vi "System.vi"(0 "Setup in":T6={"No.VI"=0, "Category"="", "StepName"="", "Seq setup flattened"="", "Comment"="", "Steps config."=[], "Jump config"=[], "Start"=0.0, "Increment"=0.0, "Name"="Pa", "Unit"="Pa", "Y data"=1, "Y prefix"="", "Y dB ref"=1.0, "Y unit"="", "Repeat State Array"=[]} {"Repeat State Array"."Start" format="%#_5g"; "Y dB ref" format="%.1f"; "Y data" items=["dB", "Lin"]; "Start" format="%#_5g"}, 5 "Data in":T4 {"Z data" items=["dB", "Lin"]; "X data" items=["dB", "Lin"]; "Y data" items=["dB", "Lin"]; "Z dB ref" format="%.1f"; "Z axis" items=["Log", "Lin"]; "X dB ref" format="%.1f"; "X axis" items=["Log", "Lin"]; "Y axis" items=["Log", "Lin"]; "Y dB ref" format="%.1f"; "Curve"."z" format="%.2f"; "Curve"."y" format="%.2f"; "Curve"."x" format="%.2f"}, 7 "Results in":T2 {"Margin" format="%.2f"}, 9 "Seq Setup in":string, 11 "Step name":string, 12 "Hardware in":string, 13 "Calibration in":string) -> (3 "Types Out":string[](array[string]), 4 "Inserted Names Out":string[](array[string]), 6 "Data out":T4 {"Z data" items=["dB", "Lin"]; "X data" items=["dB", "Lin"]; "Y data" items=["dB", "Lin"]; "Z dB ref" format="%.1f"; "Z axis" items=["Log", "Lin"]; "X dB ref" format="%.1f"; "X axis" items=["Log", "Lin"]; "Y axis" items=["Log", "Lin"]; "Y dB ref" format="%.1f"; "Curve"."z" format="%.2f"; "Curve"."y" format="%.2f"; "Curve"."x" format="%.2f"}, 8 "Results out":T2 {"Margin" format="%.2f"}, 10 "Wave out":T1[](array[typedef]) {"Y dB ref" format="%.1f"; "Y axis" items=["Log", "Lin"]; "Y data" items=["dB", "Lin"]; "X data" items=["dB", "Lin"]})   [LabVIEW 2013]
uses:
  CRYCustom and Run Seq.llb/CRYData Cluster Array.ctl
  CRYCustom and Run Seq.llb/CRYData Cluster.ctl
  CRYCustom and Run Seq.llb/CRYResult Cluster Array.ctl
  CRYCustom and Run Seq.llb/CRYResult Cluster.ctl
  CRYCustom and Run Seq.llb/CRYStep.ctl
  CRYCustom and Run Seq.llb/CRYWaveform Cluster.ctl
panel:
  in  "error in (no error)":errorcluster
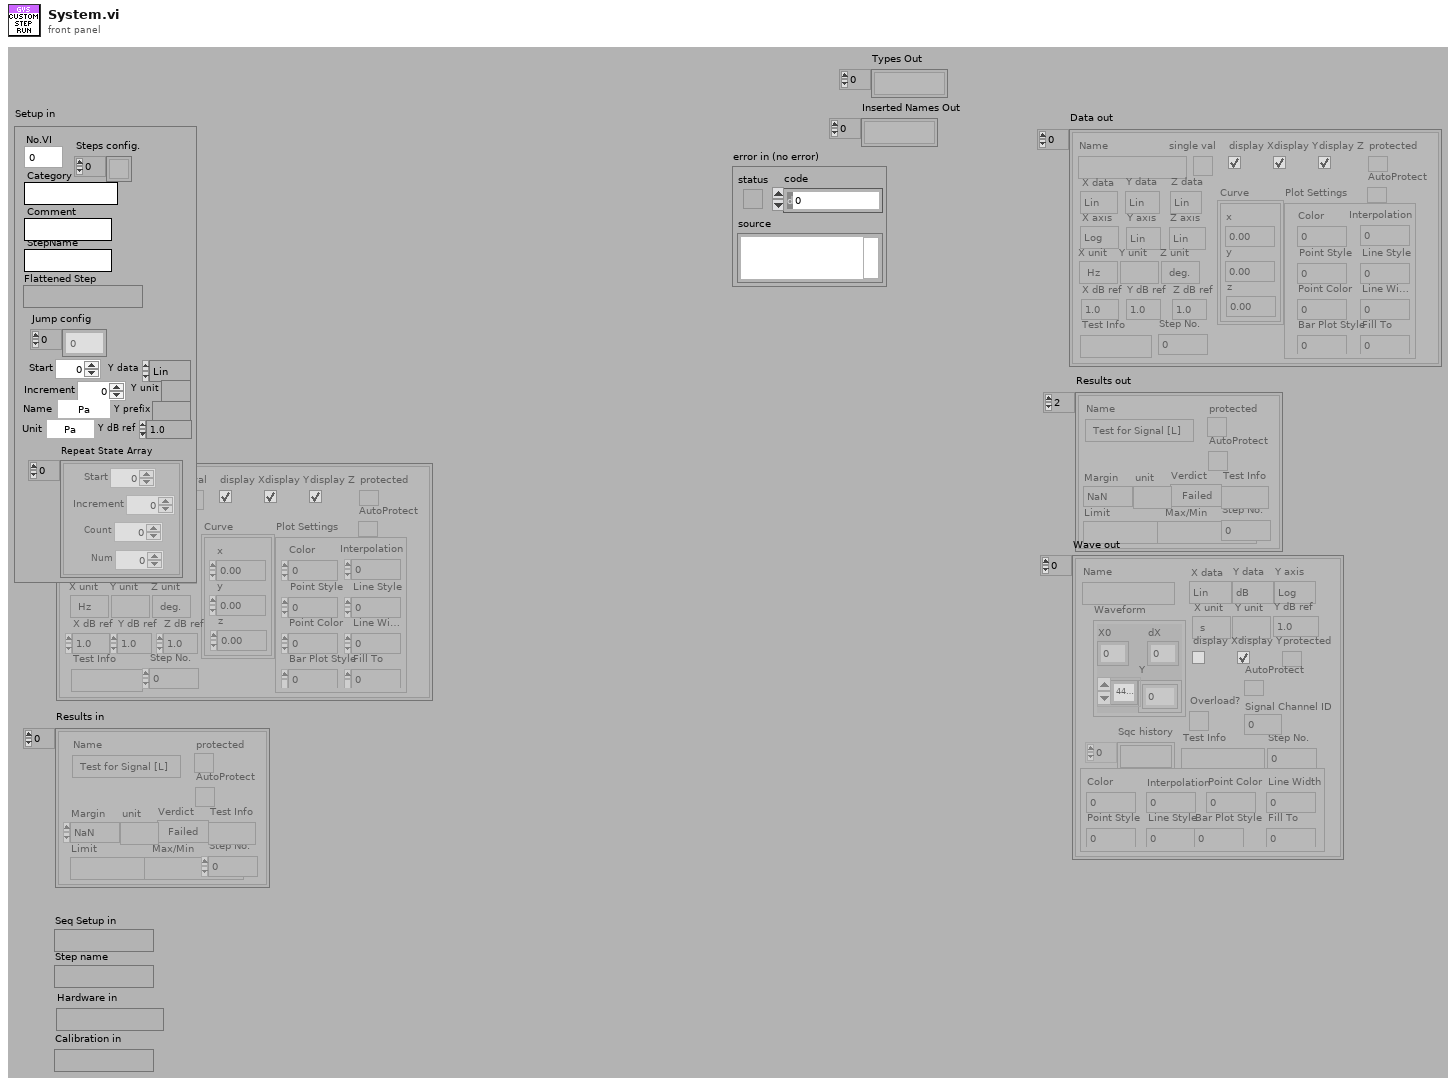
[diagram p1: front panel]
types:
  T1 = typedef "CRYWaveform Cluster.ctl" = cluster{"Waveform":cluster{"X0":dbl, "dX":dbl, "Y":sgl[]}, "X data":u16, "Y data":u16, "Y axis":u16, "X unit":string, "Y unit":string, "Y dB ref":dbl, "display Y":bool, "display X":bool, "Overload?":bool, "Test Info":string, "Step No.":i32, "Name":string, "protected":bool, "Sqc history":string[], "Signal Channel ID":i32, "Plot Settings":cluster{"Color":u32, "Interpolation":u8, "Point Style":u8, "Line Style":u8, "Point Color":u32, "Line Width":u8, "Bar Plot Style":u8, "Fill To":i16}, "AutoProtect":bool}
  T2 = typedef "CRYResult Cluster Array.ctl" = T3[]
  T3 = typedef "CRYResult Cluster.ctl" = cluster{"Name":string, "Margin":dbl, "unit":string, "Verdict":bool, "Limit":string, "Max/Min":string, "protected":bool, "Step No.":i32, "Test Info":string, "AutoProtect":bool}
  T4 = typedef "CRYData Cluster Array.ctl" = T5[]
  T5 = typedef "CRYData Cluster.ctl" = cluster{"Name":string, "Curve":cluster{"x":dbl, "y":dbl, "z":dbl}[], "X data":u16, "Y data":u16, "Z data":u16, "X axis":u16, "Y axis":u16, "Z axis":u16, "X unit":string, "Y unit":string, "Z unit":string, "X dB ref":dbl, "Y dB ref":dbl, "Z dB ref":dbl, "single val":bool, "protected":bool, "display X":bool, "display Y":bool, "display Z":bool, "Test Info":string, "Step No.":i32, "Plot Settings":cluster{"Color":u32, "Interpolation":u8, "Point Style":u8, "Line Style":u8, "Point Color":u32, "Line Width":u8, "Bar Plot Style":u8, "Fill To":i16}, "AutoProtect":bool}
  T6 = typedef "CRYStep.ctl" = cluster{"No.VI":i32, "Category":string, "StepName":string, "Seq setup flattened":string, "Comment":string, "Steps config.":bool[], "Jump config":i32[], "Start":dbl, "Increment":dbl, "Name":string, "Unit":string, "Y data":u16, "Y prefix":string, "Y dB ref":dbl, "Y unit":string, "Repeat State Array":cluster{"Start":dbl, "Increment":dbl, "Count":i32, "Num":i32}[]}
  T7 = cluster{"Command Line":string, "Working Directory":path, "WaitForCompletion":bool}
  T8 = typedef "CRYCustom Cluster.ctl" = cluster{"Help":string, "Flatten Data":string}
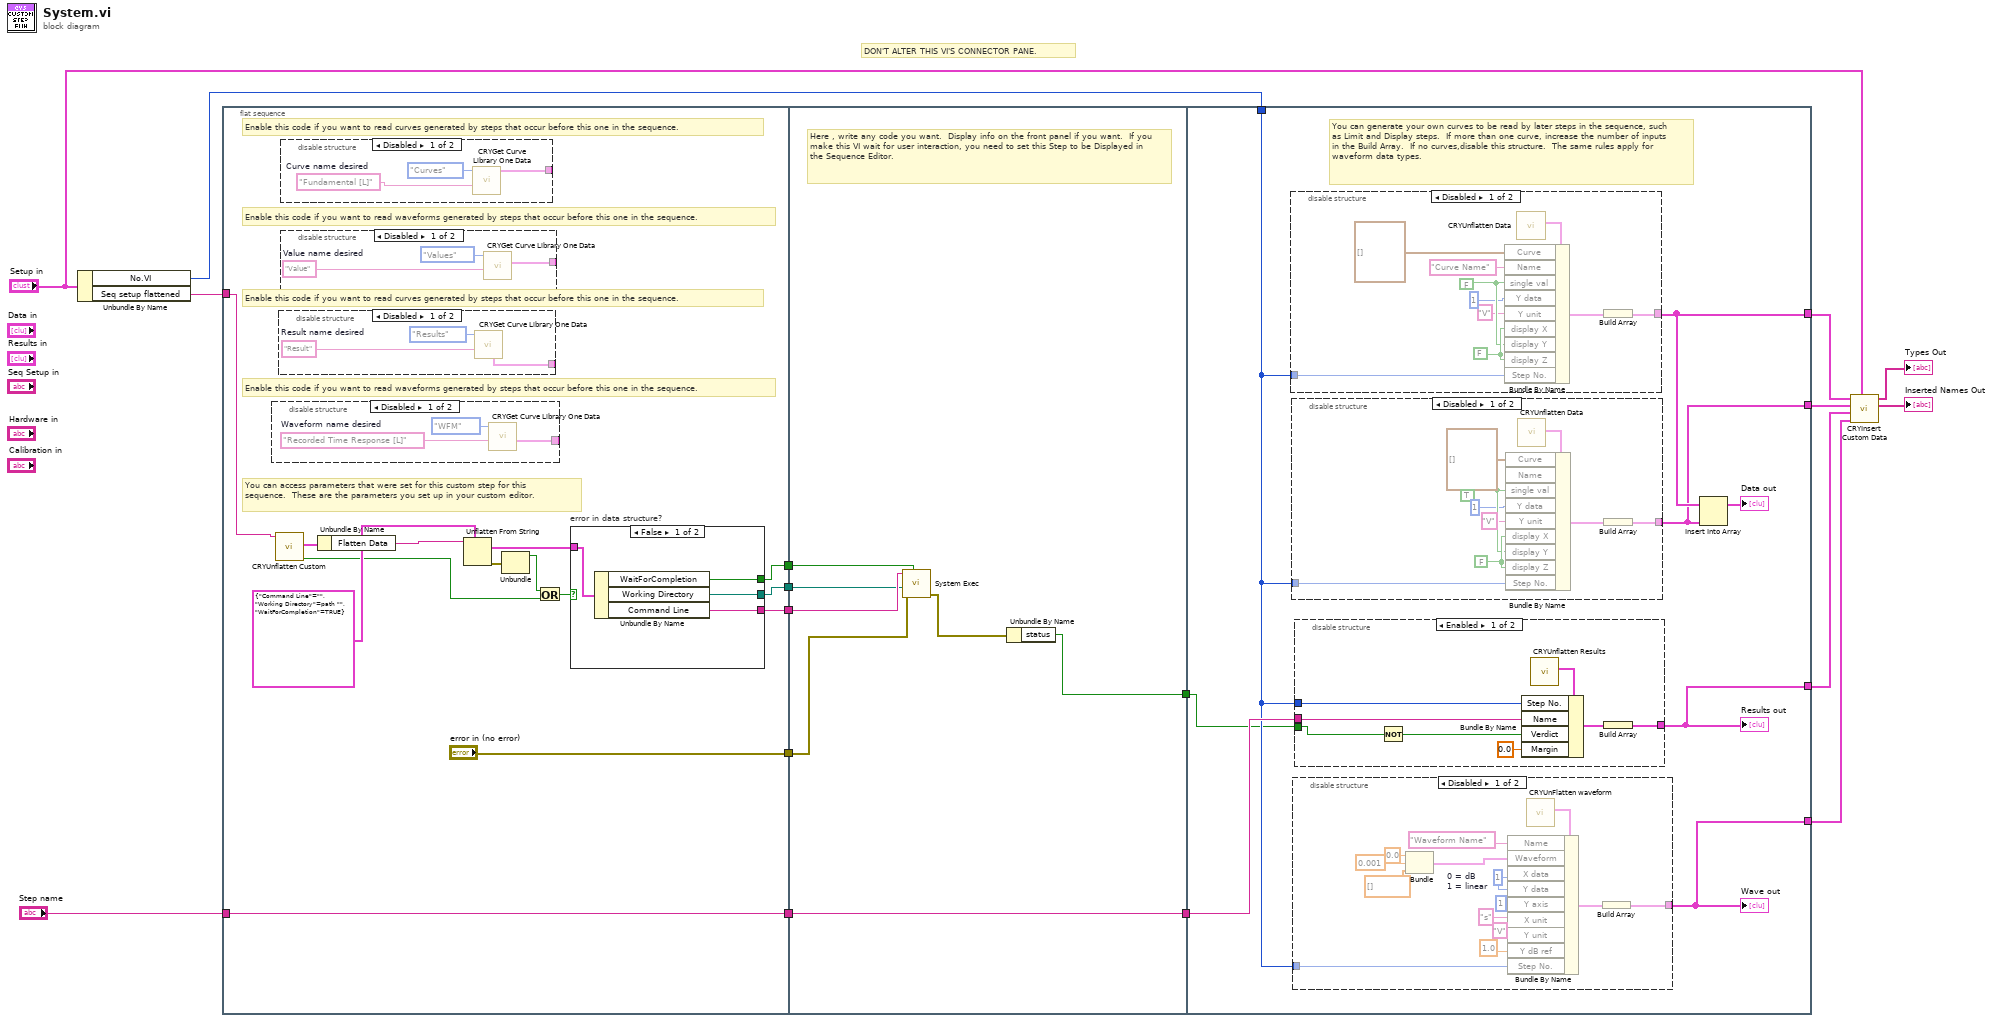
[diagram p0: block diagram]
diagram:
  # "DON'T ALTER THIS VI'S CONNECTOR PANE."
  n1 = Unbundle By Name("Setup in") -> ("No.VI"=w13:i32, "Seq setup flattened"=w17:string)
  n2 = flat-sequence {
    tunnel: w17 -> [w20]
    tunnel: "Step name" -> [w27]
    tunnel: [w27] -> w15
    tunnel: [w25] -> w5
    tunnel: [w24] -> w4
    tunnel: [w23] -> w3
    tunnel: ["error in (no error)"] -> w2
    tunnel: w15 -> [w54]
    tunnel: [w54] -> w14
    tunnel: w5 -> [w53]
    tunnel: w4 -> [w52]
    tunnel: w3 -> [w51]
    tunnel: w2 -> [w50]
    tunnel: [w49] -> w1
    tunnel: w14 -> [w62]
    tunnel: [w61] -> w10
    tunnel: [w57] -> w11
    tunnel: w13 -> [w59]
    tunnel: [w60] -> w9
    tunnel: [w58] -> w12
    tunnel: w1 -> [w55]
    frame #0 {
      # "Enable this code if you want to read waveforms generated by steps that occur before this one in the sequence."
      # "Enable this code if you want to read curves generated by steps that occur before this one in the sequence."
      # "Enable this code if you want to read waveforms generated by steps that occur before this one in the sequence."
      # "Enable this code if you want to read curves generated by steps that occur before this one in the sequence."
      # "You can access parameters that were set for this custom step for this sequence.  These are the parameters you set up in your custom editor."
      n3 = disable-structure shown="Disabled" {
        disable-tunnel: [w36 _] -> _
        frame Disabled {
          w35 = "Recorded Time Response [L]"  # Waveform name desired
          n4 = call "CRYGet Curve Library One Data .vi"("Data Name"=w35, "Type"=enum16{"Curves", "Values", "Results", "WFM"}."WFM") -> ("Wave"=w36:T1)  [unwired: 3 in, 6 out]
        }
        frame Enabled {
        }
      }
      n5 = call "CRYUnflatten Custom.vi"("Unflatten Custom"=w20) -> ("Error?"=w18:bool, "Custom"=w21:T8)  [unwired: 8 in, 1 out]
      n6 = disable-structure shown="Disabled" {
        disable-tunnel: [w32 _] -> _
        frame Disabled {
          w33 = "Result"  # Result name desired
          n7 = call "CRYGet Curve Library One Data .vi"("Data Name"=w33, "Type"=enum16{"Curves", "Values", "Results", "WFM"}."Results") -> ("Result"=w32:T3)  [unwired: 3 in, 6 out]
        }
        frame Enabled {
        }
      }
      n8 = disable-structure shown="Disabled" {
        disable-tunnel: [w38 _] -> _
        frame Disabled {
          w39 = "Fundamental [L]"  # Curve name desired
          n9 = call "CRYGet Curve Library One Data .vi"("Data Name"=w39, "Type"=enum16{"Curves", "Values", "Results", "WFM"}."Curves") -> ("Curve"=w38:T5)  [unwired: 3 in, 6 out]
        }
        frame Enabled {
        }
      }
      n10 = disable-structure shown="Disabled" {
        disable-tunnel: [w41 _] -> _
        frame Disabled {
          w42 = "Value"  # Value name desired
          n11 = call "CRYGet Curve Library One Data .vi"("Data Name"=w42, "Type"=enum16{"Curves", "Values", "Results", "WFM"}."Values") -> ("Value"=w41:T5)  [unwired: 3 in, 6 out]
        }
        frame Enabled {
        }
      }
      n12 = Unbundle By Name(w21) -> ("Flatten Data"=w19:string)
      n13 = Unflatten From String(type=T7 {"Command Line"="", "Working Directory"=path "", "WaitForCompletion"=TRUE}, binary string=w19) -> (value=w30:T7, error out=w31:errorcluster)  [unwired: 1 in, 3 out]
      n14 = Unbundle(w31) -> ("status"=w28:bool)  [unwired: 2 out]
      n15 = Or(x=w28, y=w18) -> (x .or. y?=w29:bool)
      n16 = case "error in data structure?" shown="False" w29 {
        tunnel: w30 -> [w47 _]
        tunnel: [w46 _] -> w25
        tunnel: [w45 _] -> w23
        tunnel: [w44 _] -> w24
        frame False {
          n17 = Unbundle By Name(w47) -> ("WaitForCompletion"=w46:bool, "Working Directory"=w45:path, "Command Line"=w44:string)
        }
        frame True {
        }
      }
    }
    frame #1 {
      # "Here , write any code you want.  Display info on the front panel if you want.  If you make this VI wait for user interaction, you need to set this Step to be Displayed in the Sequence Editor."
      n18 = call <vilib>:"System Exec.vi"("wait until completion? (T)"=w53, "error in (no error)"=w50, "working directory"=w51, "command line"=w52) -> ("error out"=w48:errorcluster)  [unwired: 2 in, 5 out]
      n19 = Unbundle By Name(w48) -> ("status"=w49:bool)
    }
    frame #2 {
      # "You can generate your own curves to be read by later steps in the sequence, such as Limit and Display steps.  If more than one curve, increase the number of inputs in the Build Array.  If no curves,disable this structure.  The same rules apply for waveform data types."
      n20 = disable-structure shown="Disabled" {
        disable-tunnel: w59 -> [w68 _]
        disable-tunnel: [w63 _] -> w58
        frame Disabled {
          w71 = FALSE
          w70 = FALSE
          n21 = call "CRYUnflatten Data.vi"() -> ("Datum"=w72:T5)  [unwired: 9 in, 2 out]
          n22 = Bundle By Name(cluster=w72, "Curve"=cluster{"x":dbl, "y":dbl, "z":dbl}[] [] ("appended array"), "Name"="Curve Name", "single val"=w70, "Y data"=u16 1, "Y unit"="V", "display X"=w71, "display Y"=w70, "display Z"=w71, "Step No."=w68) -> (w64:T5)
          n23 = Build Array(w64) -> (w63:T5[])
        }
        frame Enabled {
        }
      }
      n24 = disable-structure shown="Disabled" {
        disable-tunnel: w59 -> [w77 _]
        disable-tunnel: [w75 _] -> w57
        frame Disabled {
          w80 = FALSE
          w79 = TRUE
          n25 = call "CRYUnflatten Data.vi"() -> ("Datum"=w81:T5)  [unwired: 9 in, 2 out]
          n26 = Bundle By Name(cluster=w81, "Curve"=cluster{"x":dbl, "y":dbl, "z":dbl}[] [], "single val"=w79, "Y data"=u16 1, "Y unit"="V", "display X"=w80, "display Y"=w79, "display Z"=w80, "Step No."=w77) -> (w76:T5)  [unwired: 1 in]
          n27 = Build Array(w76) -> (w75:T5[])
        }
        frame Enabled {
        }
      }
      n28 = disable-structure shown="Disabled" {
        disable-tunnel: [w91 _] -> w60
        disable-tunnel: w59 -> [w90 _]
        frame Disabled {
          w96 = u16 1  # 0 = dB 1 = linear
          n29 = Bundle ("Actual waveform data bundle.\nX0\ndX\n[Y] array")(0.0, 0.001, dbl[] []) -> (w100:cluster{dbl, dbl, dbl[]})  [unwired: 1 out]
          n30 = call "CRYUnFlatten waveform.vi"() -> ("Waveform Cluster"=w101:T1)  [unwired: 9 in, 2 out]
          n31 = Bundle By Name(cluster=w101, "Name"="Waveform Name" ("Bundle Element"), "Waveform"=w100, "X data"=w96, "Y data"=w96, "Y axis"=u16 1, "X unit"="s", "Y unit"="V", "Y dB ref"=1.0, "Step No."=w90) -> (w102:T1)
          n32 = Build Array(w102) -> (w91:T1[])
        }
        frame Enabled {
        }
      }
      "Wave out" <- w60
      n33 = disable-structure shown="Enabled" {
        disable-tunnel: w59 -> [w87 _]
        disable-tunnel: w62 -> [w86 _]
        disable-tunnel: [w85 _] -> w61
        disable-tunnel: w55 -> [w84 _]
        frame Enabled {
          n34 = Not(x=w84) -> (.not. x?=w83:bool)
          n35 = call "CRYUnflatten Results.vi"() -> ("Result"=w88:T3)  [unwired: 9 in, 2 out]
          n36 = Bundle By Name(cluster=w88, "Step No."=w87, "Name"=w86, "Verdict"=w83, "Margin"=0.0) -> (w89:T3)
          n37 = Build Array(w89) -> (w85:T3[])
        }
        frame Disabled {
        }
      }
      "Results out" <- w61
      n38 = Insert Into Array(array=w58, new element=w57) -> (→"Data out":T5[])  [unwired: 1 in]
    }
  }
  n39 = call "CRYInsert Custom Data.vi"("Setup in"="Setup in", "Wave"=w9, "Results"=w10, "Values"=w11, "Curves"=w12) -> ("Inserted Names Out"=→"Inserted Names Out":string[], "Types Out"=→"Types Out":string[])  [unwired: 5 in]
